vi "Write Setpoint.vi"(8 "error in":errorcluster, 10 "Setpoint":sgl, 11 "Alicat Device in":refnum<class "Alicat Device.lvclass">) -> (0 "error out":errorcluster, 2 "DataOut":string, 3 "Alicat Device out":refnum<class "Alicat Device.lvclass">)   [LabVIEW 2018, in "Alicat Lib.lvlib" / "Alicat Device.lvclass"]
doc: "Send a command to the controller for the setpoint. The command will be in the format <b>Xnnnnn</b> where <b>X</b> is the address and <b>nnnnn</b> is a setpoint value that ranges from 0 to 64000. The setpoint is based on the <b>Fullscale</b> value and can be calculated as\n\nnnnnn = SP*64000/FS\n\nWhen the command for a new setpoint is sent, the controller will respond with the current data values. The input <b>Setpoint</b> will be coerced in the range 0 to Full Scale."
uses:
  Alicat Device.lvclass
  C:/Users/Labview/Documents/exscalabar_server/Devices/Configurable Device/Configurable Device.lvclass
  Alicat Device.lvclass/Alicat Device.ctl
  Configurable Device/Configurable Device.lvclass/Configurable Device.ctl
  Configurable Device/Read Log Session.vi
  Configurable Device/Read ID.vi
  Configurable Device/Read controller_.vi
  reusable/Session APIs/Serial/Public/Get Data/Get String.vi
  <userlib>/_Session Fwk/Session - Root.lvclass
  reusable/Session APIs/Serial/Serial Session.lvclass
  reusable/Session APIs/Session Log/System Log.lvclass
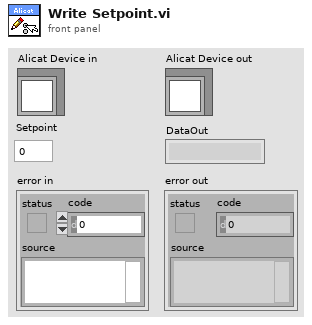
[diagram p1: front panel]
types:
  T1 = typedef "Serial Session.lvclass/Session Handle.ctl" = refnum<data-value>
  T2 = typedef "Session - Root.lvclass/Session Handle.ctl" = refnum<data-value>
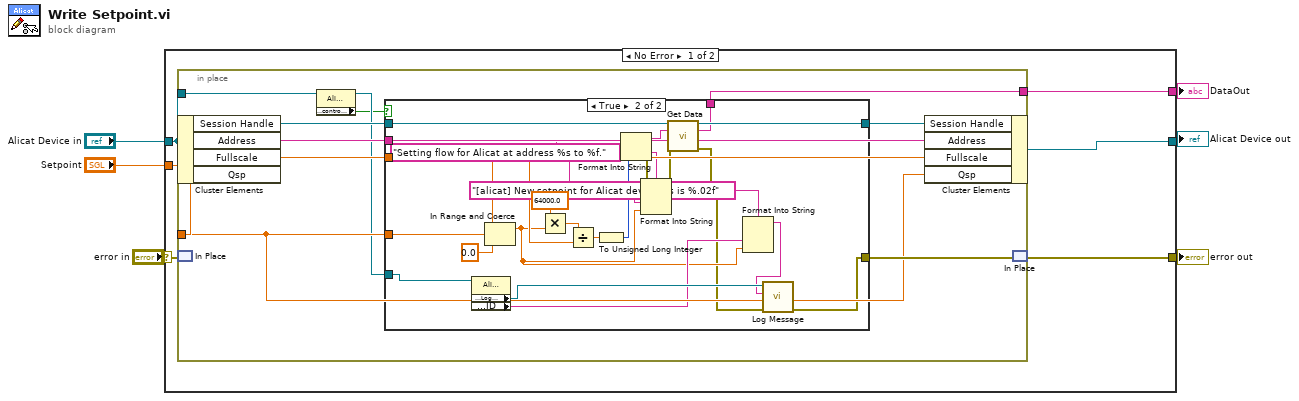
[diagram p0: block diagram]
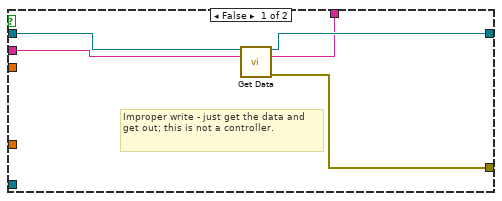
[diagram p2: hidden frame]
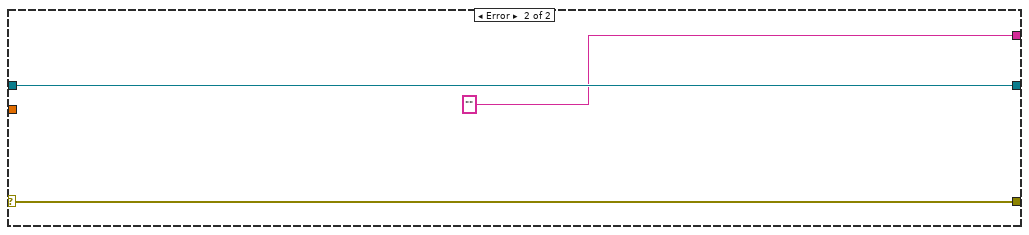
[diagram p3: hidden frame]
diagram:
  n1 = case shown="No Error" "error in" {
    selector: "error in" -> [w12 w53]
    tunnel: "Alicat Device in" -> [w7 w52]
    tunnel: [w10 w53] -> w2
    tunnel: [w11 w52] -> w3
    tunnel: [w9 "" ("DataOut")] -> w4
    tunnel: "Setpoint" -> [w8 _]
    frame No Error {
      n2 = in-place {
        in-place-border: [w19] -> w9
        in-place-border: w8 -> [w16]
        in-place-border: w7 -> [w15]
        n3 = in-place-cluster #1(w7) -> ("Session Handle"=w22:T1, "Address"=w18:string, "Fullscale"=w17:sgl)  [unwired: 1 out]
        n4 = in-place-match #2(w12) -> ()  [unwired: 1 out]
        n5 = property class="Alicat Device"(reference=w15) -> (reference out=w14:refnum<class "Alicat Device.lvclass">, "Accessors:controller_"=w13:bool)  [unwired: 1 in, 1 out]
        n6 = case shown="True" w13 {
          tunnel: w22 -> [w26 w50]
          tunnel: [w25 w49] -> w21
          tunnel: [w23 w28] -> w20
          tunnel: [w24 w48] -> w19
          tunnel: w18 -> [w27 w39]
          tunnel: w17 -> [_ w42]
          tunnel: w16 -> [_ w40]
          tunnel: w14 -> [_ w35]
          frame False {
            # "Improper write - just get the data and get out; this is not a controller."
            n7 = call-poly "Get Data.vi"("Session Handle in"=w26, "CMD"=w27) -> ("Session Handle out"=w25:T1, "DataOut"=w24:string, "error out"=w23:errorcluster)  [unwired: 11 in]
          }
          frame True {
            n8 = property class="Alicat Device"(reference=w35) -> ("Accessors:Log Session"=w34:T2, "Accessors:ID"=w32:string)  [unwired: 1 in, 2 out]
            n9 = In Range and Coerce(upper limit=w42, x=w40, lower limit=sgl 0.0) -> (coerced(x)=w31:sgl)  [unwired: 1 out]
            n10 = Multiply(x=sgl 64000.0, y=w31) -> (x*y=w46:sgl)
            n11 = Divide(x=w46, y=w42) -> (x/y=w45:sgl)
            n12 = To Unsigned Long Integer(number=w45) -> (unsigned 32bit integer=w43:u32)
            n13 = Format Into String(initial string=w39, w43) -> (resulting string=w47:string, error out=w36:errorcluster)  [unwired: 2 in]
            n14 = Format Into String(format string="Setting flow for Alicat at address %s to %f.", error in=w36, w39, w31) -> (error out=w37:errorcluster)  [unwired: 1 in, 1 out]
            n15 = call-poly "Get Data.vi"("Session Handle in"=w50, "CMD"=w47, "error in"=w37) -> ("Session Handle out"=w49:T1, "DataOut"=w48:string, "error out"=w29:errorcluster)  [unwired: 10 in]
            n16 = Format Into String(format string="[alicat] New setpoint for Alicat device %s is %.02f", w32, w31) -> (resulting string=w30:string)  [unwired: 2 in, 1 out]
            n17 = call "Log Message.vi"("error in"=w29, "MSG In"=w30, "session in"=w34) -> ("error out"=w28:errorcluster)  [unwired: 7 in, 1 out]
          }
        }
        n18 = in-place-cluster #1("Session Handle"=w21, "Address"=w18, "Fullscale"=w17, "Qsp"=w16) -> (w11:refnum<class "Alicat Device.lvclass">)
        n19 = in-place-match #2(w20) -> (w10:errorcluster)
      }
    }
    frame Error {
    }
  }
  "error out" <- w2
  "Alicat Device out" <- w3
  "DataOut" <- w4
